vi "Lead Durability.vi"() -> ()   [LabVIEW 2013]
uses:
  <vilib>/Instr/_visa.llb/VISA Configure Serial Port (Serial Instr).vi
  <vilib>/Utility/file.llb/Write To Spreadsheet File (string).vi
panel:
  in  "Filename Note":string
  in  "Stop if fail":bool=TRUE
  in  "Array":string[](array[string])
  in  "Reset 11":bool
  in  "Reset 10":bool
  in  "Reset 9":bool
  in  "Reset 8":bool
  in  "Reset 7":bool
  in  "Reset 6":bool
  in  "Reset 5":bool
  in  "Reset 4":bool
  in  "Reset 3":bool
  in  "Reset 2":bool
  in  "Reset 1":bool
  in  "Reset 0":bool
  out "green":i32[](array[numeric])
  out "Waveform Graph":i32[][](graph)
  in  "Play Button":bool
  out "Lead Contact":bool[](array[boolean])
  out "error out":errorcluster
  out "accel":string
  in  "Angle":dbl=180.0 min=0.0 max=350.0 step=5.0
  out "concatenated string 2":string
  out "concatenated string":string
  in  "Hz":dbl=2.0 min=0.25 max=2.5 step=0.25
  in  "stop":bool
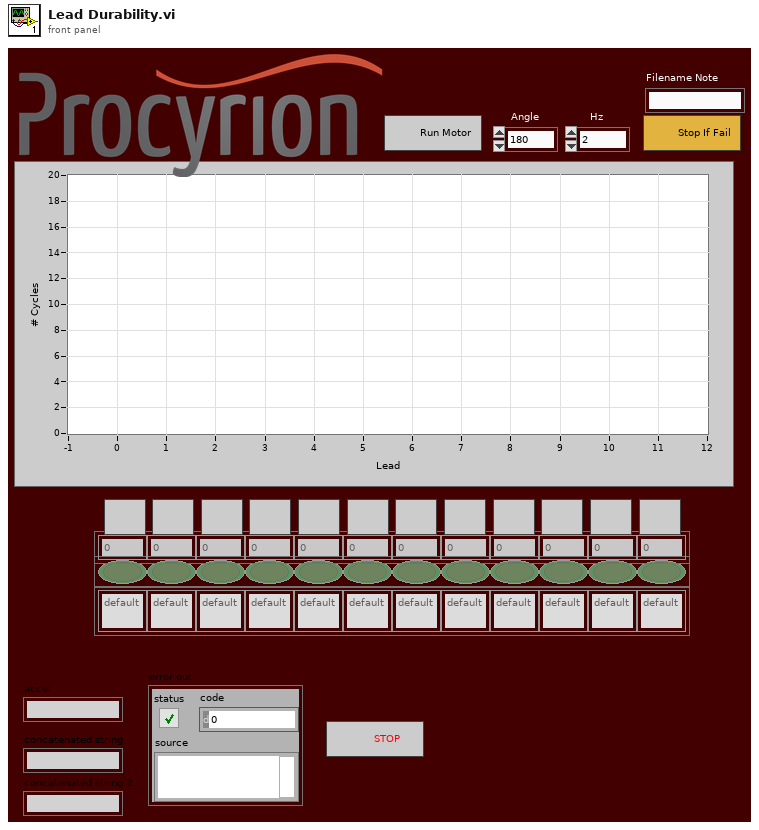
[diagram p1: front panel]
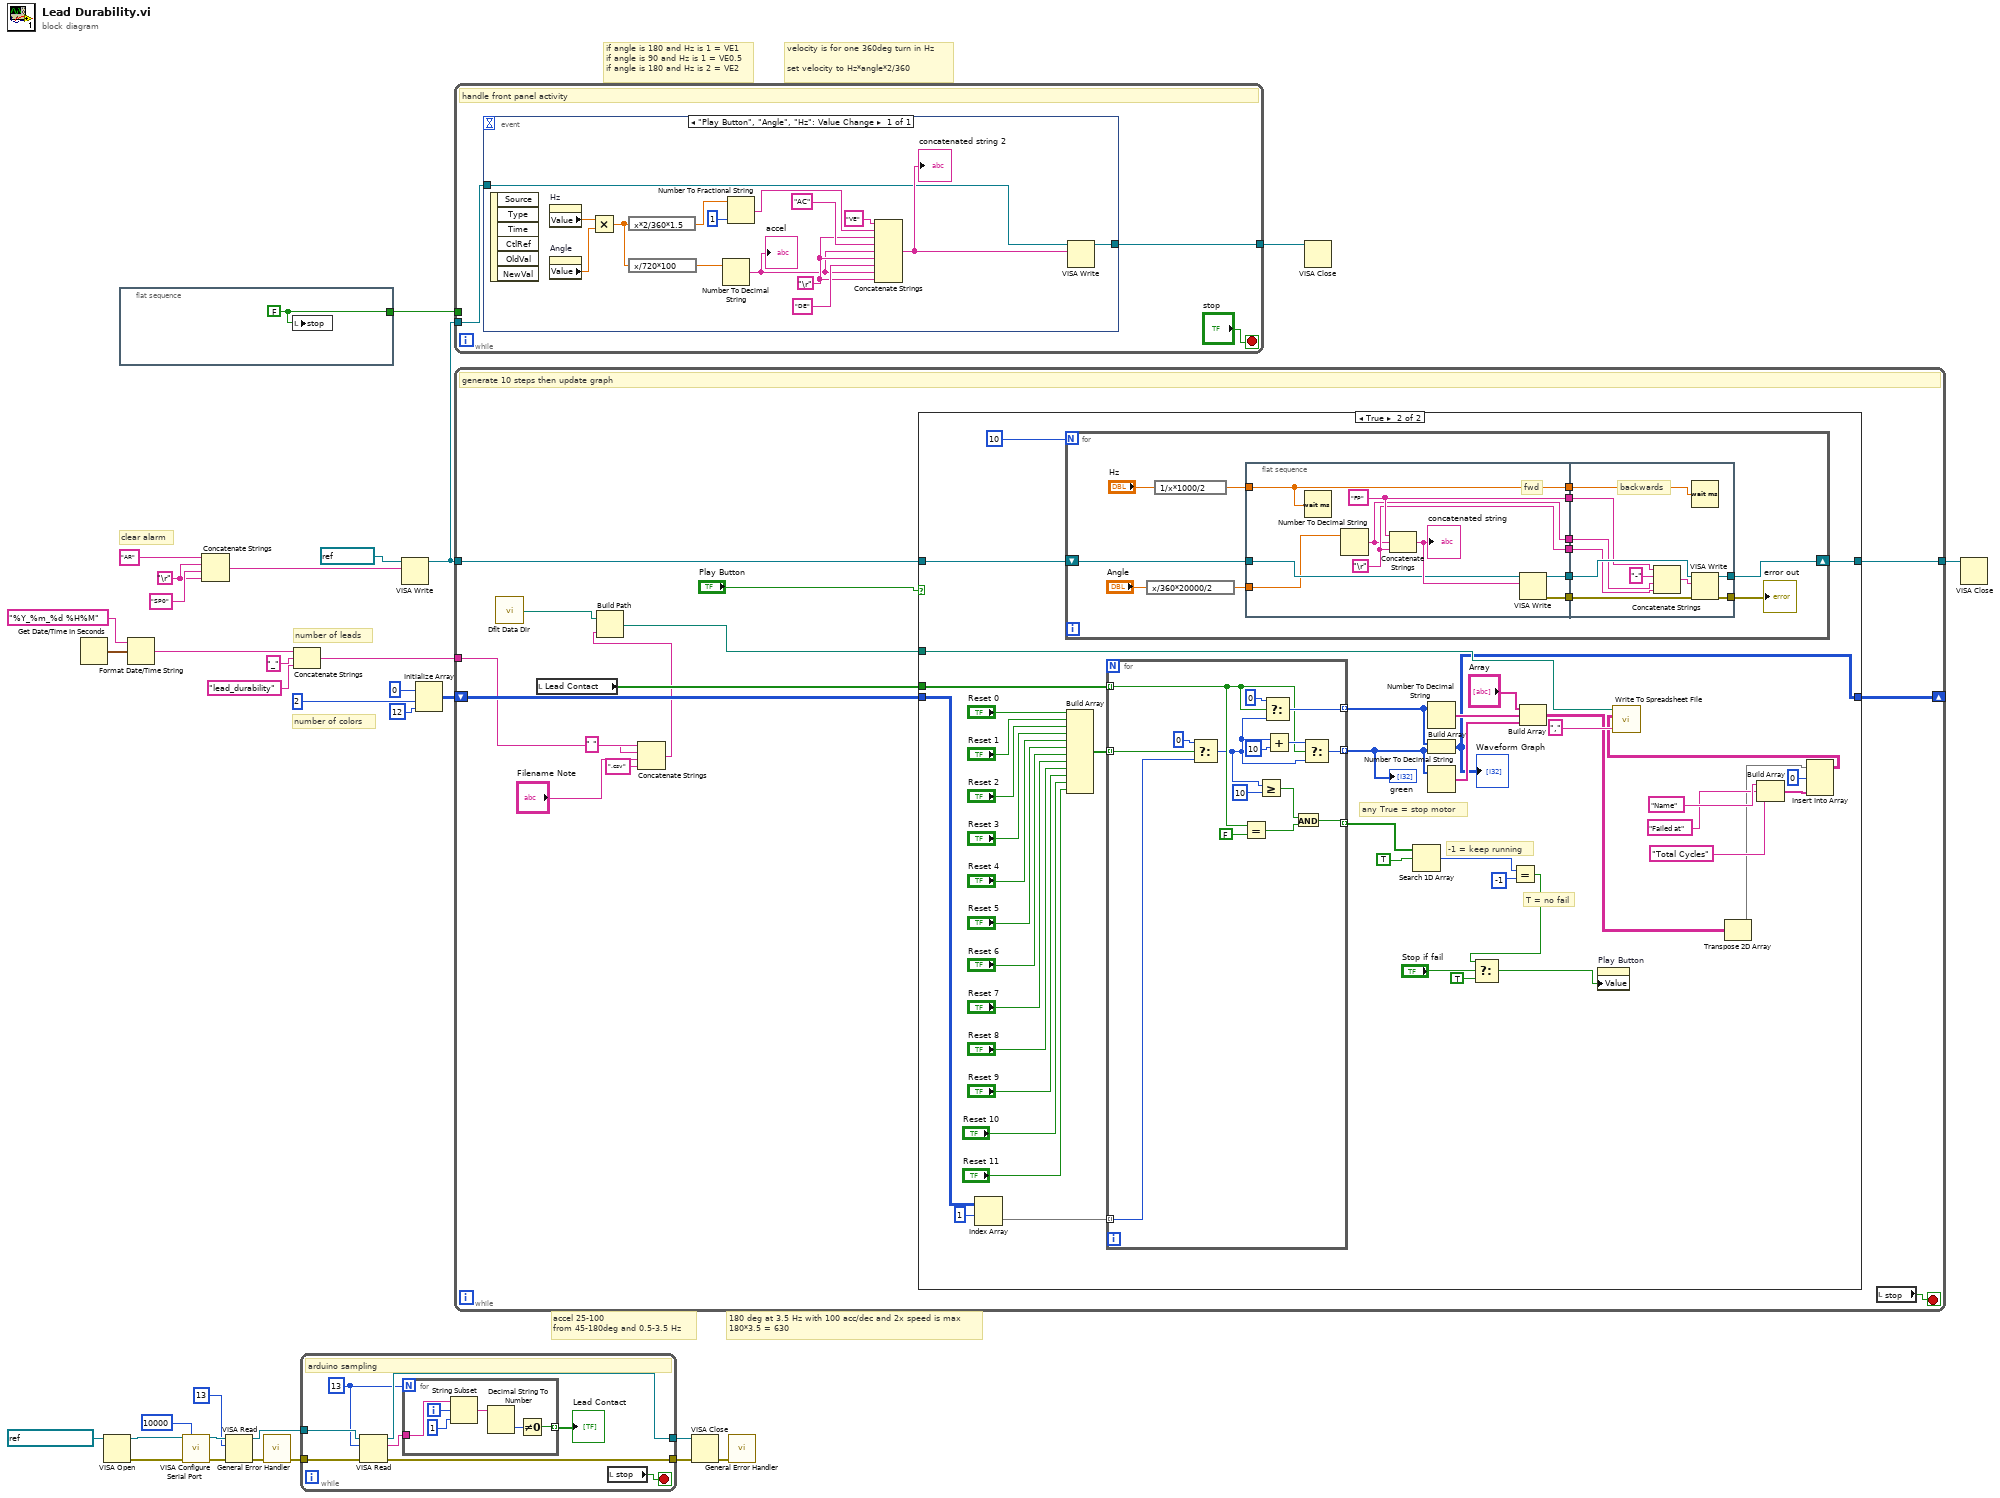
[diagram p0: block diagram]
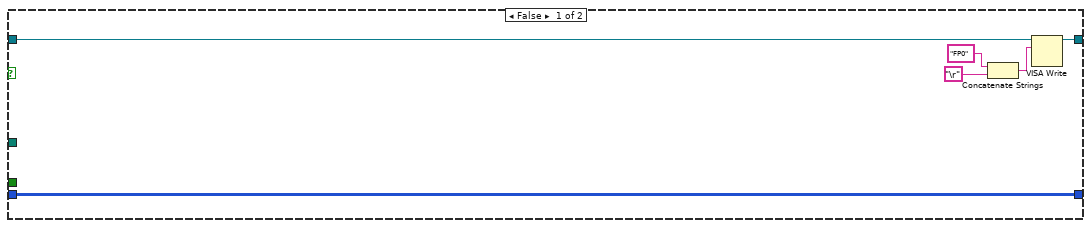
[diagram p2: hidden frame]
diagram:
  w28 = "\r"
  # "number of colors"
  # "number of leads"
  # "180 deg at 3.5 Hz with 100 acc/dec and 2x speed is max\n180*3.5 = 630"
  # "accel 25-100\nfrom 45-180deg and 0.5-3.5 Hz"
  # "if angle is 180 and Hz is 1 = VE1\nif angle is 90 and Hz is 1 = VE0.5\nif angle is 180 and Hz is 2 = VE2"
  # "velocity is for one 360deg turn in Hz\n\nset velocity to Hz*angle*2/360"
  # "clear alarm"
  n1 = Get Date/Time In Seconds() -> (seconds since 1Jan1904=w9:timestamp)
  n2 = VISA Open(VISA resource name=refnum<visa-resource-name> "ASRL8::INSTR" ("VISA resource")) -> (VISA resource name=w3:refnum<visa-resource-name>, error out=w2:errorcluster)  [unwired: 4 in]
  n3 = flat-sequence {
    tunnel: [w33] -> w24
    frame #0 {
      w33 = FALSE ("stop")
      n4 = local write "stop"(w33) -> ()
    }
  }
  n5 = Format Date/Time String(time format string (%c)="%Y_%m_%d %H%M", seconds (now)=w9) -> (date/time string=w6:string)  [unwired: 1 in]
  n6 = call-poly "VISA Configure Serial Port"("VISA resource name"=w3, "timeout (10sec)"=u32 10000, "error in (no error)"=w2) -> ("VISA resource name out"=w15:refnum<visa-resource-name>, "error out"=w14:errorcluster)  [unwired: 11 in]
  n7 = Concatenate Strings("AR" ("write buffer"), w28, "SP0" ("write buffer"), w28) -> (w31:string)
  n8 = VISA Read(VISA resource name=w15, byte count=u32 13, error in (no error)=w14) -> (VISA resource name out=w13:refnum<visa-resource-name>, error out=w12:errorcluster)  [unwired: 2 out]
  n9 = call <vilib>:"General Error Handler.vi"("error in (no error)"=w12) -> ("error out"=w5:errorcluster)  [unwired: 10 in, 4 out]
  n10 = Concatenate Strings(w6, "_", "lead_durability" ("string")) -> (w1:string)
  n11 = while {
    tunnel: w13 -> [w39]
    tunnel: [w38] -> w19
    tunnel: w5 -> [w37]
    tunnel: [w34] -> w18
    stop <- w41 stop-if-true
    w35 = u32 13 ("byte count")
    # "arduino sampling"
    n12 = VISA Read(VISA resource name=w39, byte count=w35, error in (no error)=w37) -> (VISA resource name out=w38:refnum<visa-resource-name>, read buffer=w36:string, error out=w34:errorcluster)  [unwired: 1 out]
    n13 = for {
      N: w35 -> [_]
      tunnel: [w42] -> w40 mode=indexing
      tunnel: w36 -> [w47]
      i -> [w46]
      n14 = String Subset(string=w47, offset (0)=w46, length (rest)=1 ("length (rest)")) -> (substring=w44:string)
      n15 = Decimal String To Number(string=w44) -> (number=w43:i32)  [unwired: 2 in, 1 out]
      n16 = Not Equal To 0?(x=w43) -> (x != 0?=w42:bool)
    }
    "Lead Contact" <- w40
    n17 = local read "stop"() -> (w41:bool)
  }
  n18 = VISA Write(VISA resource name=refnum<visa-resource-name> "COM4", write buffer=w31) -> (VISA resource name out=w27:refnum<visa-resource-name>)  [unwired: 1 in, 2 out]
  n19 = Initialize Array(0, 2 ("dimension size"), 12 ("dimension size")) -> (w20:i32[][])
  n20 = while {
    tunnel: w27 -> [w49]
    tunnel: [w48] -> w25
    tunnel: w24 -> [_]
    stop <- "stop" stop-if-true
    # "handle front panel activity"
    n21 = event shown="[0] \"Play Button\", \"Angle\", \"Hz\": Value Change" {
      selector: _ -> [_]
      dyn-events: _ -> [_]
      timeout: _ -> [_]
      tunnel: w49 -> [w60]
      tunnel: [w51] -> w48
      event "Play Button", "Angle", "Hz": Value Change {
        w55 = "\r"
        n22 = event-data() -> ()  [unwired: 1 in, 6 out]
        n23 = property on="Hz" class="DigNum (strict)"() -> ("Value"=w53:dbl)  [unwired: 2 in, 2 out]
        n24 = property on="Angle" class="DigNum (strict)"() -> ("Value"=w52:dbl)  [unwired: 2 in, 2 out]
        n25 = Multiply(x=w53, y=w52) -> (x*y=w58:dbl)
        n26 = expression code="x*2/360*1.5"(w58) -> (w65:dbl)
        n27 = expression code="x/720*100"(w58) -> (w57:dbl)
        n28 = Number To Decimal String(number=w57) -> (decimal integer string=w54:string)  [unwired: 1 in]
        "accel" <- w54
        n29 = Number To Fractional String(number=w65, precision (6)=i16 1) -> (F-format string=w64:string)  [unwired: 2 in]
        n30 = Concatenate Strings("VE" ("write buffer"), w64, w55, "AC" ("write buffer"), w54, w55, "DE" ("write buffer"), w54, w55) -> (w61:string)
        "concatenated string 2" <- w61
        n31 = VISA Write(VISA resource name=w60, write buffer=w61) -> (VISA resource name out=w51:refnum<visa-resource-name>)  [unwired: 1 in, 2 out]
      }
    }
  }
  n32 = while {
    tunnel: w27 -> [w78]
    tunnel: [w79] -> w26
    shift-right: [w76] -> _
    shift-left: w20 -> [w74]
    tunnel: w1 -> [w71]
    stop <- w77 stop-if-true
    # "generate 10 steps then update graph"
    n33 = call <vilib>:"Dflt Data Dir.vi"() -> ("App:Default Data Directory"=w72:path)
    n34 = local read "Lead Contact"() -> (w75:bool[])
    n35 = Concatenate Strings(w71, " " ("string"), "Filename Note", ".csv" ("string")) -> (w67:string)
    n36 = Build Path(base path=w72, name or relative path=w67) -> (appended path=w66:path)
    n37 = case shown="True" "Play Button" {
      tunnel: [w83 w129] -> w79
      tunnel: w78 -> [w84 w128]
      tunnel: w75 -> [_ w126]
      tunnel: [w85 w104] -> w76
      tunnel: w74 -> [w85 w124]
      tunnel: w66 -> [_ w109]
      frame False {
        n38 = Concatenate Strings("FP0" ("write buffer"), "\r") -> (w80:string)
        n39 = VISA Write(VISA resource name=w84, write buffer=w80) -> (VISA resource name out=w83:refnum<visa-resource-name>)  [unwired: 1 in, 2 out]
      }
      frame True {
        # "-1 = keep running"
        # "any True = stop motor"
        # "T = no fail"
        n40 = Index Array(array=w124, index (row)=1) -> (element=w123:i32[])  [unwired: 1 in]
        n41 = for {
          N: 10 -> [_]
          shift-right: [w153] -> w129
          shift-left: w128 -> [w150]
          n42 = expression code="x/360*20000/2"("Angle") -> (w145:dbl)
          n43 = expression code="1/x*1000/2"("Hz") -> (w156:dbl)
          n44 = flat-sequence {
            tunnel: w156 -> [w166]
            tunnel: [w166] -> w155
            tunnel: w145 -> [w163]
            tunnel: w150 -> [w164]
            tunnel: [w162] -> w154
            tunnel: [w161] -> w151
            tunnel: [w160] -> w149
            tunnel: [w159] -> w148
            tunnel: [w158] -> w147
            tunnel: w155 -> [w176]
            tunnel: w154 -> [w175]
            tunnel: [w174] -> w153
            tunnel: [w173] -> w152
            tunnel: w151 -> [w172]
            tunnel: w149 -> [w171]
            tunnel: w148 -> [w170]
            tunnel: w147 -> [w169]
            frame #0 {
              w159 = "\r"
              w160 = "FP" ("write buffer")
              # "fwd"
              n45 = Wait (ms)(milliseconds to wait=w166) -> ()  [unwired: 1 out]
              n46 = Number To Decimal String(number=w163) -> (decimal integer string=w158:string)  [unwired: 1 in]
              n47 = Concatenate Strings(w160, w158, w159) -> (w165:string)
              "concatenated string" <- w165
              n48 = VISA Write(VISA resource name=w164, write buffer=w165) -> (VISA resource name out=w162:refnum<visa-resource-name>, error out=w161:errorcluster)  [unwired: 1 in, 1 out]
            }
            frame #1 {
              # "backwards"
              n49 = Concatenate Strings(w171, "-" ("string"), w169, w170) -> (w167:string)
              n50 = Wait (ms)(milliseconds to wait=w176) -> ()  [unwired: 1 out]
              n51 = VISA Write(VISA resource name=w175, write buffer=w167, error in (no error)=w172) -> (VISA resource name out=w174:refnum<visa-resource-name>, error out=w173:errorcluster)  [unwired: 1 out]
            }
          }
          "error out" <- w152
        }
        n52 = Build Array("Reset 0", "Reset 1", "Reset 2", "Reset 3", "Reset 4", "Reset 5", "Reset 6", "Reset 7", "Reset 8", "Reset 9", "Reset 10", "Reset 11") -> (w110:bool[])
        n53 = for {
          tunnel: w126 -> [w136] mode=indexing
          tunnel: w123 -> [w138] mode=indexing
          tunnel: [w143] -> w105 mode=indexing
          tunnel: [w141] -> w106 mode=indexing
          tunnel: w110 -> [w139] mode=indexing
          tunnel: [w130] -> w101 mode=indexing
          n54 = Select(t=0, s=w139, f=w138) -> (s? t:f=w134:i32)
          n55 = Equal?(x=w136, y=FALSE) -> (x = y?=w131:bool)
          n56 = Greater Or Equal?(x=w134, y=10) -> (x >= y?=w132:bool)
          n57 = Select(t=0, s=w136, f=w134) -> (s? t:f=w141:i32)
          n58 = Add(x=w134, y=10) -> (x+y=w144:i32)
          n59 = And(x=w132, y=w131) -> (x .and. y?=w130:bool)
          n60 = Select(t=w144, s=w136, f=w134) -> (s? t:f=w143:i32)
        }
        "green" <- w105
        n61 = Search 1D Array(1D array=w101, element=TRUE) -> (index of element=w99:i32)  [unwired: 1 in]
        n62 = Number To Decimal String(number=w106) -> (decimal integer string=w108:string[])  [unwired: 1 in]
        n63 = Build Array(w106, w105) -> (w104:i32[][])
        "Waveform Graph" <- w104
        n64 = Number To Decimal String(number=w105) -> (decimal integer string=w107:string[])  [unwired: 1 in]
        n65 = Equal?(x=w99, y=-1) -> (x = y?=w97:bool)
        n66 = Select(t=w97, s="Stop if fail", f=TRUE) -> (s? t:f=w95:bool)
        n67 = Build Array("Array", w108, w107) -> (w87:string[][])
        n68 = property on="Play Button" class="Bool (strict)"("Value"=w95) -> ()  [unwired: 2 in, 2 out]
        n69 = Transpose 2D Array(2D array=w87) -> (transposed array=w86:string[][])
        n70 = Build Array("Name", "Failed at", "Total Cycles") -> (w89:string[])
        n71 = Insert Into Array(array=w86, index (row)=0 ("index"), new element=w89) -> (w88:string[][])  [unwired: 1 in]
        n72 = call-poly <vilib>:"Write To Spreadsheet File.vi"("delimiter (\\t)"="," ("delimiter (\\t)"), "2D data"=w88, "file path (dialog if empty)"=w109) -> ()  [unwired: 5 in, 1 out]
      }
    }
    n73 = local read "stop"() -> (w77:bool)
  }
  n74 = VISA Close(VISA resource name=w19, error in (no error)=w18) -> (error out=w17:errorcluster)
  n75 = call <vilib>:"General Error Handler.vi"("error in (no error)"=w17) -> ()  [unwired: 10 in, 5 out]
  n76 = VISA Close(VISA resource name=w25) -> ()  [unwired: 1 in, 1 out]
  n77 = VISA Close(VISA resource name=w26) -> ()  [unwired: 1 in, 1 out]
